vi "Action.vi"(8 "error in (no error)":errorcluster, 10 "OOQMH in":refnum<class "OOQMH.lvclass">, 11 "Stop in":refnum<class "Stop.lvclass">) -> (0 "error out":errorcluster, 2 "OOQMH out":refnum<class "OOQMH.lvclass">, 3 "Stop out":refnum<class "Stop.lvclass">)   [LabVIEW 2024, in "OOQMH.lvlib" / "Stop.lvclass"]
uses:
  Stop.lvclass
  OOQMH/OOQMH.lvclass
  Stop.lvclass/Stop.ctl
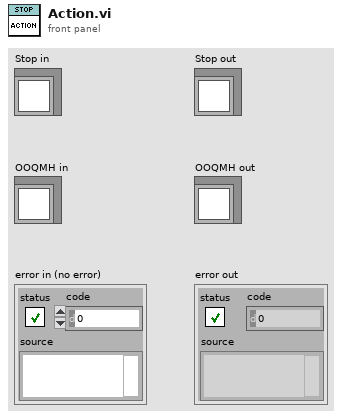
[diagram p1: front panel]
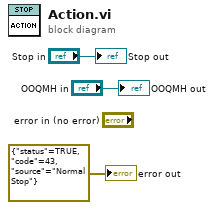
[diagram p0: block diagram]
diagram:
  "error out" <- errorcluster {"status"=TRUE, "code"=43, "source"="Normal Stop"} ("error out")
  "Stop out" <- "Stop in"
  "OOQMH out" <- "OOQMH in"
